vi "tsdb_set_signal_value_can.vi"(6 "SigValue":dbl, 7 "Signal Str":string, 8 "错误输入（无错误）":errorcluster, 9 "Message":string, 10 "CAN ObJ":T1, 11 "path":path) -> (0 "错误输出":errorcluster, 1 "return":i32, 2 "CANObJ":T1, 3 "path out":path)   [LabVIEW 2014]
doc: "Function Introduction :\nSet the CANFD insulation signal based on the Message name and signal name\nCall location :\nAfter loading the database, this function can be called from any location (application connection status, disconnected status)\nNumber.\ninput parameter :\nACANFD: CANFD message (reference)\nAMsgName: Message Name\nASgnName: Signal Name\nAValue: Signal value\nReturn value :\n==0: Execution successful\nOther values: Query error code"
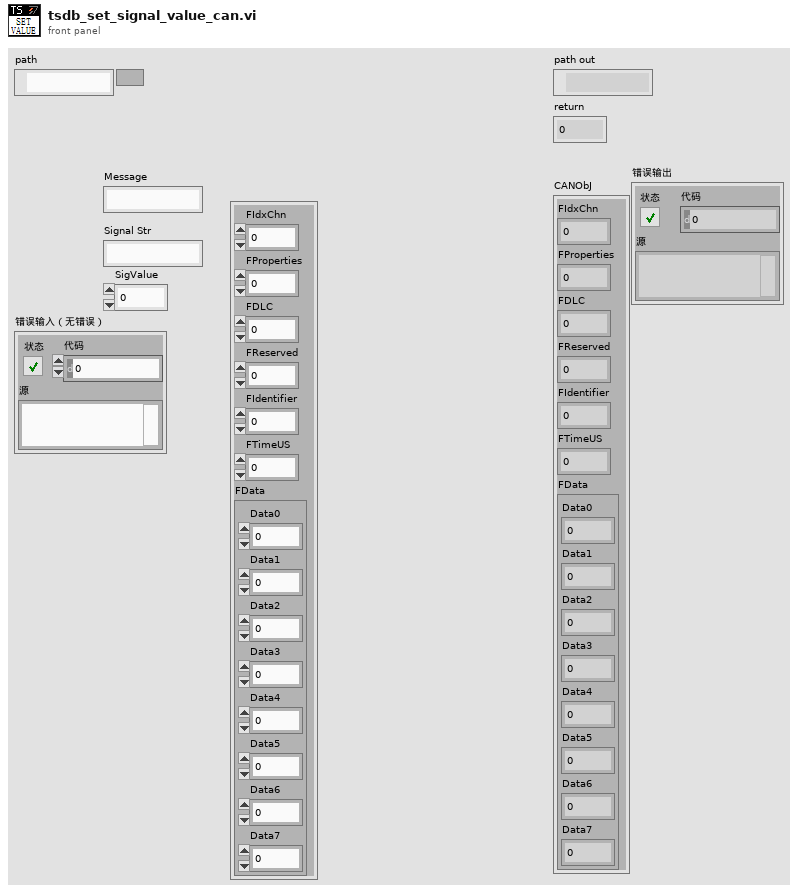
[diagram p1: front panel]
types:
  T1 = cluster{"FIdxChn":u8, "FProperties":u8, "FDLC":u8, "FReserved":u8, "FIdentifier":i32, "FTimeUS":u64, "FData":cluster{"Data0":u8, "Data1":u8, "Data2":u8, "Data3":u8, "Data4":u8, "Data5":u8, "Data6":u8, "Data7":u8}}
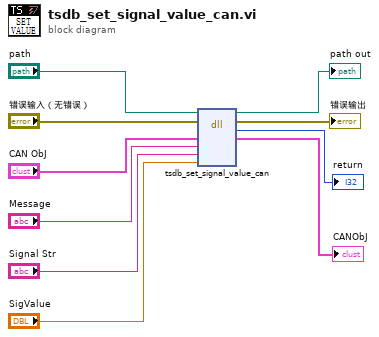
[diagram p0: block diagram]
diagram:
  n1 = dll-call lib="D:/Program Files (x86)/TOSUN/TSMaster/bin/TSMaster.dll" fn="tsdb_set_signal_value_can"(path in="path", error in="错误输入（无错误）", "CANObJ"="CAN ObJ", "Message"="Message", "Signal"="Signal Str", "SigValue"="SigValue") -> (path out=→"path out":path, error out=→"错误输出":errorcluster, "tsdb_get_signal_value_can"=→"return":i32, "CANObJ"=→"CANObJ":T1)  [unwired: 4 in]
